vi "PLCtoGUIBoolArray.vi"(9 "Read Size":i32, 11 "DB Input Vals":u8[](array[numeric])=[0, 0, 0, 0]) -> (2 "array":bool[](array[boolean]))   [LabVIEW 2023]
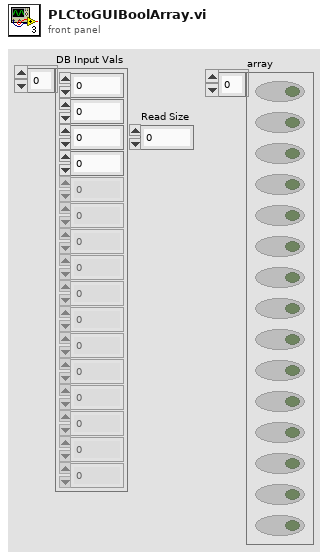
[diagram p1: front panel]
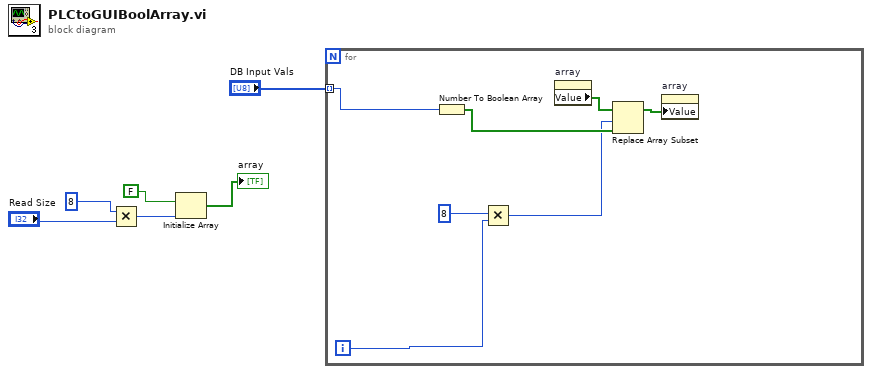
[diagram p0: block diagram]
diagram:
  n1 = Multiply(x=8, y="Read Size") -> (x*y=w3:i32)
  n2 = Initialize Array(FALSE, w3) -> (→"array":bool[])
  n3 = for {
    tunnel: "DB Input Vals" -> [w13] mode=indexing
    i -> [w8]
    n4 = Number To Boolean Array(number=w13) -> (Boolean array=w10:bool[])
    n5 = Multiply(x=8, y=w8) -> (x*y=w7:i32)
    n6 = property on="array" class="Arr (strict)"() -> ("Value"=w12:bool[])  [unwired: 2 in, 2 out]
    n7 = Replace Array Subset(array=w12, new element=w10, index=w7) -> (w11:bool[])
    n8 = property on="array" class="Arr (strict)"("Value"=w11) -> ()  [unwired: 2 in, 2 out]
  }
